vi "Unitary_Test_Start.vi"() -> (0 "Test_passed":bool)   [LabVIEW 2015]
panel:
  out "hidden 2":errorcluster
  out "error 2 must falil":errorcluster
  out "hidden3 2":errorcluster
  in  "Experience ID1 2":string="TestBAD"
  out "error 1 must be OK":errorcluster
  out "hidden3":errorcluster
  out "hidden":errorcluster={"status"=TRUE, "code"=1149, "source"="Invoke Node in close.vi->Unitary_Test_Start.vi\n<APPEND>\nMethod Name: <b>Front Panel:Close</b>"}
  in  "Experience ID1":string="TestOK"
  out "Test_OK":bool[](array[boolean])=[TRUE, FALSE]
  # "Test basic methods with some testing plant"
  # "This test take time because a vi refuses to close\n(its part of the test)"
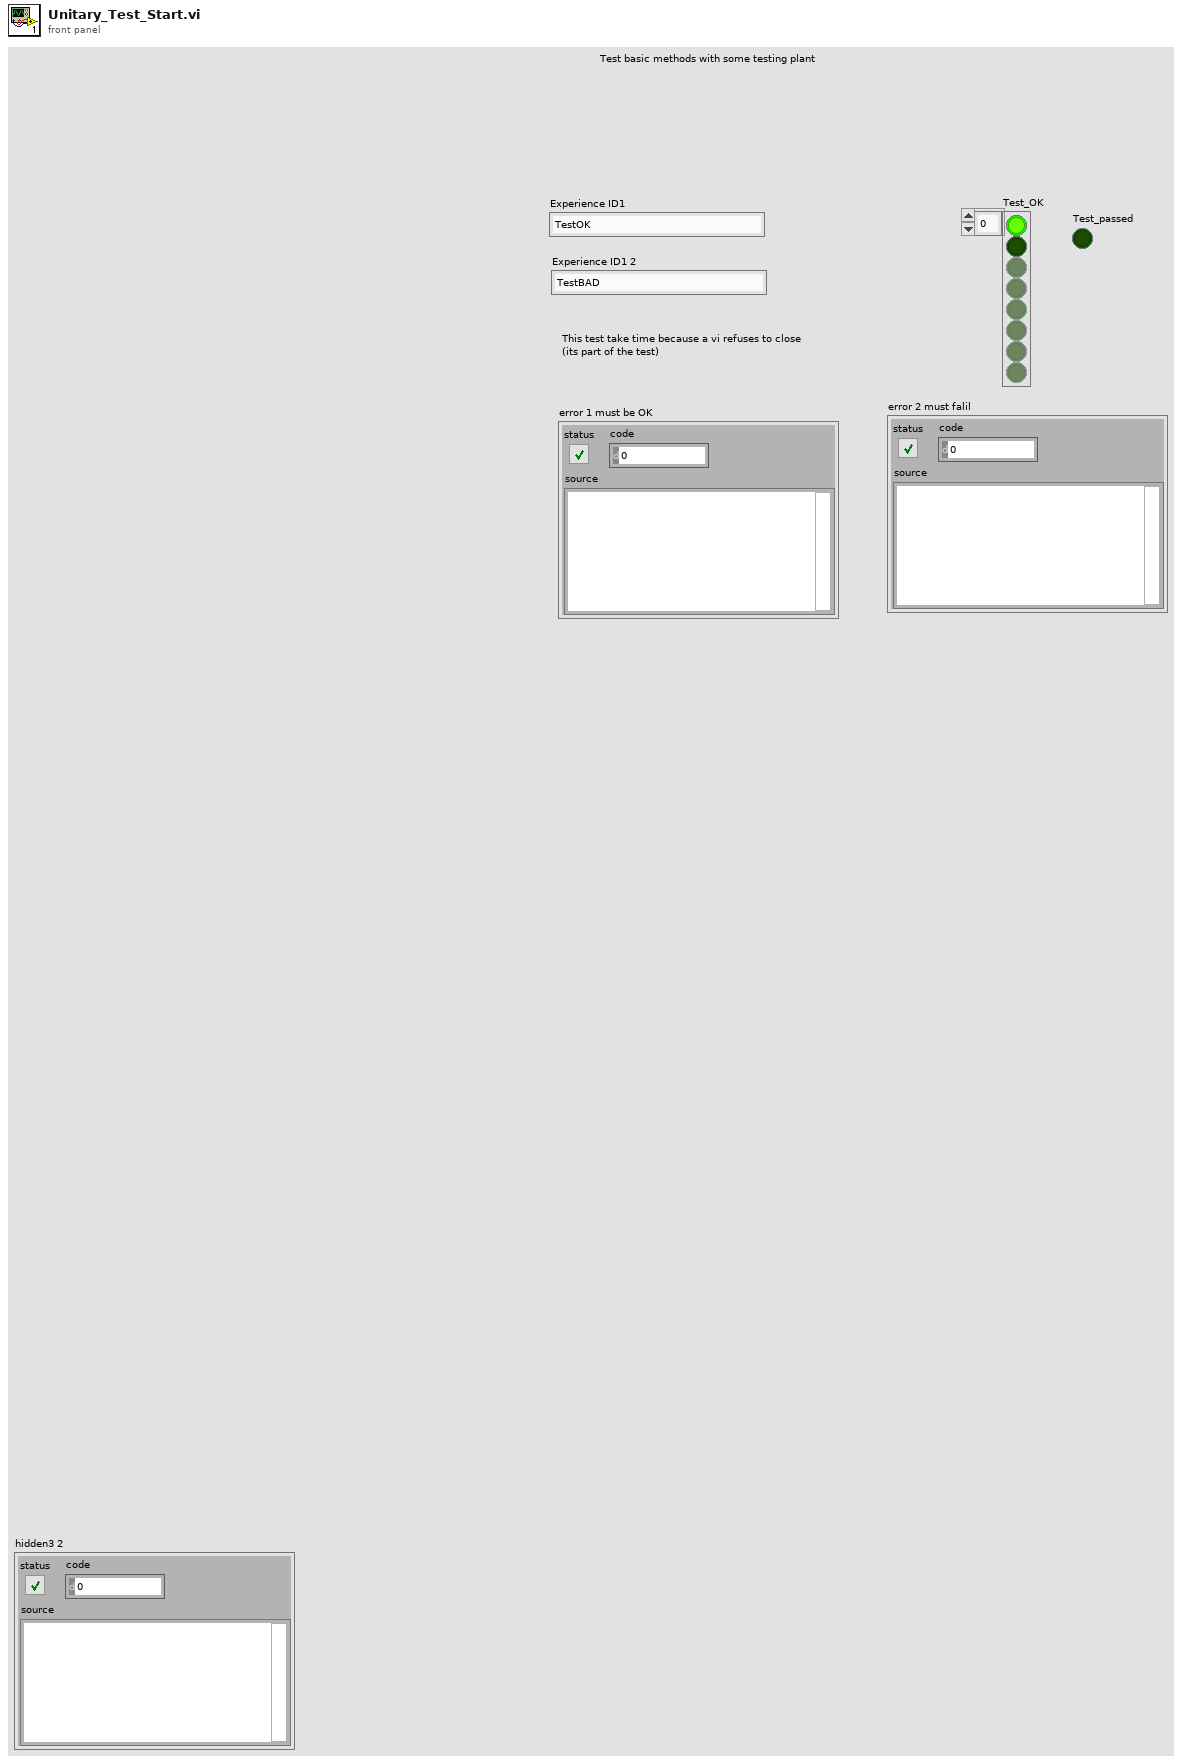
[diagram p1: front panel]
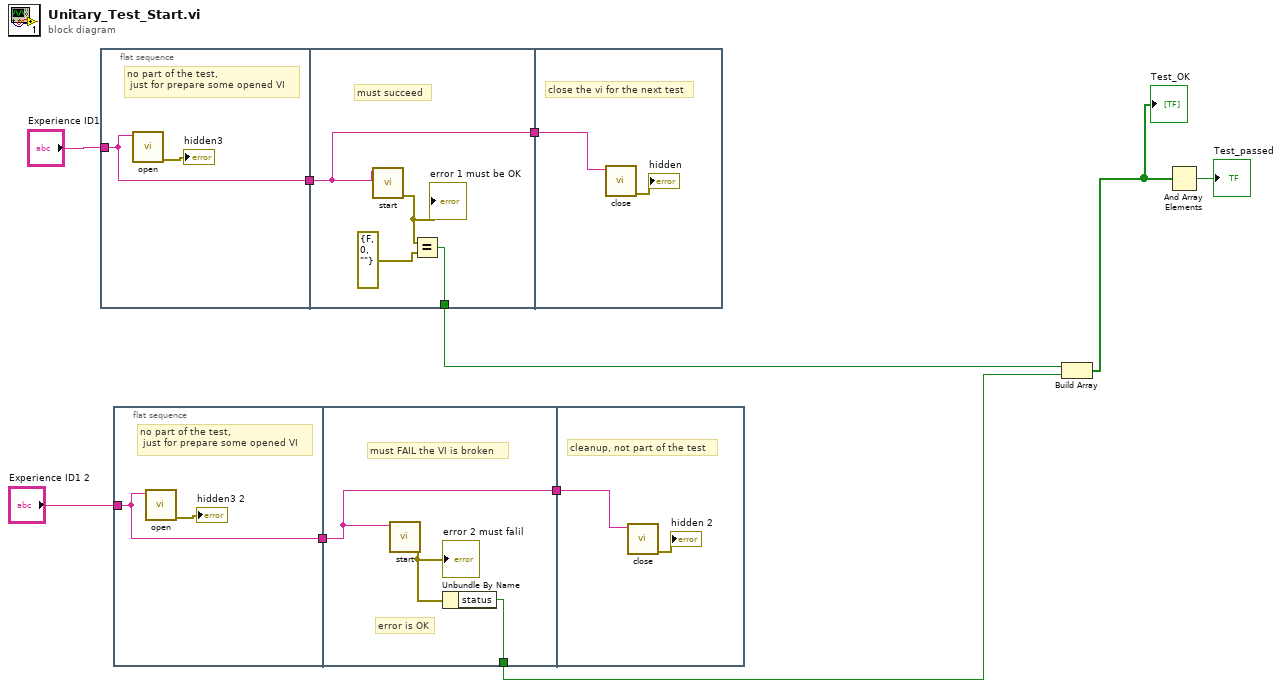
[diagram p0: block diagram]
diagram:
  n1 = flat-sequence {
    tunnel: "Experience ID1" -> [w12]
    tunnel: [w12] -> w2
    tunnel: w2 -> [w14]
    tunnel: [w14] -> w7
    tunnel: [w15] -> w8
    tunnel: w7 -> [w17]
    frame #0 {
      # "no part of the test,\n just for prepare some opened VI"
      n2 = call "open.vi"("Experience ID"=w12) -> ("error out"=→"hidden3":errorcluster)  [unwired: 8 in, 2 out]
    }
    frame #1 {
      # "must succeed"
      n3 = call "start.vi"("Experience ID"=w14) -> ("error out"=w13:errorcluster)  [unwired: 10 in]
      "error 1 must be OK" <- w13
      n4 = Equal?(x=w13, y=errorcluster {"status"=FALSE, "code"=0, "source"=""} ("error out")) -> (x = y?=w15:bool)
    }
    frame #2 {
      # "close the vi for the next test"
      n5 = call "close.vi"("Experience ID"=w17) -> ("error out"=→"hidden":errorcluster)  [unwired: 10 in]
    }
  }
  n6 = flat-sequence {
    tunnel: "Experience ID1 2" -> [w20]
    tunnel: [w20] -> w1
    tunnel: w1 -> [w22]
    tunnel: [w22] -> w5
    tunnel: [w23] -> w3
    tunnel: w5 -> [w24]
    frame #0 {
      # "no part of the test,\n just for prepare some opened VI"
      n7 = call "open.vi"("Experience ID"=w20) -> ("error out"=→"hidden3 2":errorcluster)  [unwired: 8 in, 2 out]
    }
    frame #1 {
      # "error is OK"
      # "must FAIL the VI is broken"
      n8 = call "start.vi"("Experience ID"=w22) -> ("error out"=w21:errorcluster)  [unwired: 10 in]
      "error 2 must falil" <- w21
      n9 = Unbundle By Name(w21) -> ("status"=w23:bool)
    }
    frame #2 {
      # "cleanup, not part of the test"
      n10 = call "close.vi"("Experience ID"=w24) -> ("error out"=→"hidden 2":errorcluster)  [unwired: 10 in]
    }
  }
  n11 = Build Array(w8, w3) -> (w6:bool[])
  "Test_OK" <- w6
  n12 = And Array Elements(Boolean array=w6) -> (logical AND=→"Test_passed":bool)
